vi "robotFearBall.vi"(6 "Robot in":refnum<class "Robot.lvclass">, 7 "Raio":dbl=123.0, 8 "error in (no error)":errorcluster, 9 "Game":refnum<class "Game.lvclass">, 10 "Target":dbl[](array[numeric]), 11 "KickToSkill in":refnum<class "KickToSkill.lvclass">) -> (0 "error out":errorcluster, 2 "Robot out":refnum<class "Robot.lvclass">, 3 "KickToSkill out":refnum<class "KickToSkill.lvclass">)   [LabVIEW 2021, in "KickToSkill.lvclass"]
uses:
  KickToSkill.lvclass
  Robot_class/Robot.lvclass
  Game_class/Game.lvclass
  Game_class/Game.lvclass/Game.ctl
  Object_class/Object.lvclass/Object.ctl
  Robot_class/Robot.lvclass/Robot.ctl
  Game_class/Read BallRef.vi
  Object_class/Read position(x,y).vi
  Robot_class/Write dest_x.vi
  Robot_class/Write dest_y.vi
  Robot_class/Write dest_orientation.vi
  Ball_class/Ball.lvclass
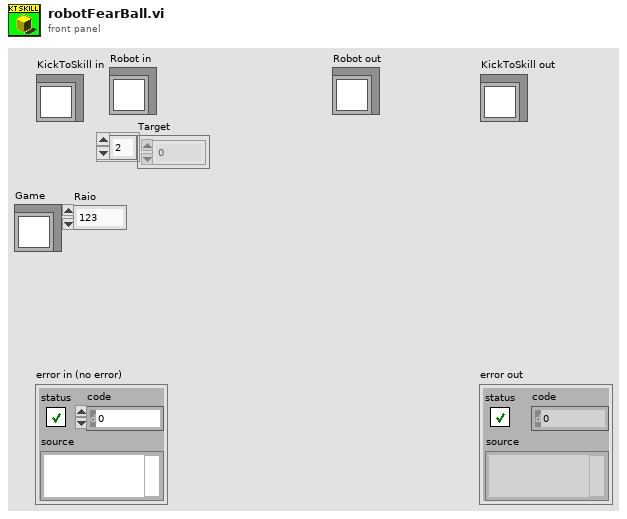
[diagram p1: front panel]
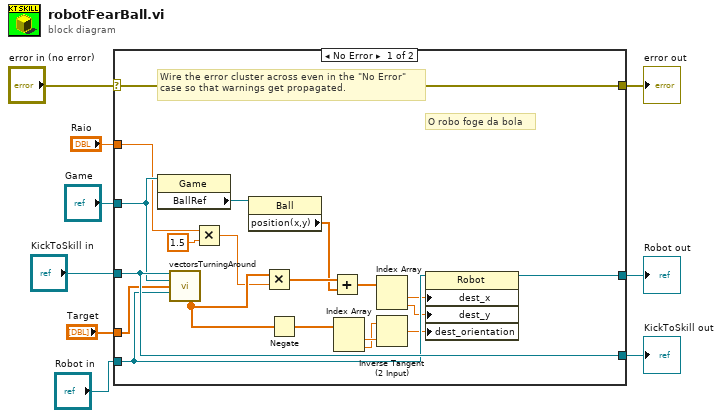
[diagram p0: block diagram]
diagram:
  n1 = case shown="No Error" "error in (no error)" {
    selector: "error in (no error)" -> [w29 w32]
    tunnel: [w29 w32] -> w8
    tunnel: [w28 w31] -> w6
    tunnel: "KickToSkill in" -> [w28 w31]
    tunnel: "Robot in" -> [w22 w30]
    tunnel: [w21 w30] -> w4
    tunnel: "Raio" -> [w12 _]
    tunnel: "Game" -> [w26 _]
    tunnel: "Target" -> [w27 _]
    frame No Error {
      # "O robo foge da bola"
      # "Wire the error cluster across even in the \"No Error\"\ncase so that warnings get propagated."
      n2 = property class="Game"(reference=w26) -> ("BallRef"=w25:refnum<class "Ball.lvclass">)  [unwired: 1 in, 2 out]
      n3 = call "vectorsTurningAround.vi"("KickToSkill in"=w28, "Game"=w26, "Target"=w27, "Robot in"=w22) -> ("R-B"=w17:dbl[])  [unwired: 4 in, 7 out]
      n4 = Multiply(x=w12, y=1.5) -> (x*y=w11:dbl)
      n5 = property class="Ball"(reference=w25) -> ("position(x,y)"=w23:dbl[])  [unwired: 1 in, 2 out]
      n6 = Multiply(x=w17, y=w11) -> (x*y=w24:dbl[])
      n7 = Negate(x=w17) -> (-x=w16:dbl[])
      n8 = Add(x=w24, y=w23) -> (x+y=w20:dbl[])
      n9 = Index Array(array=w16) -> (element #1=w15:dbl, element #2=w14:dbl)  [unwired: 2 in]
      n10 = Index Array(array=w20) -> (element #1=w19:dbl, element #2=w18:dbl)  [unwired: 2 in]
      n11 = Inverse Tangent (2 Input)(1:w15, 2:w14) -> (0:w13:dbl)
      n12 = property class="Robot"(reference=w22, "dest_x"=w19, "dest_y"=w18, "dest_orientation"=w13) -> (reference out=w21:refnum<class "Robot.lvclass">)  [unwired: 1 in, 1 out]
    }
    frame Error {
    }
  }
  "error out" <- w8
  "KickToSkill out" <- w6
  "Robot out" <- w4
